vi "Command Intake Cube.vi"(7 "Startup":bool, 9 "Timeout":u32, 11 "Speed":dbl) -> (3 "Output":dbl, 4 "Reinit":bool, 6 "Completed":bool)   [LabVIEW 2017]
uses:
  Command Execution State.ctl
  Intake/Intake Globals.vi
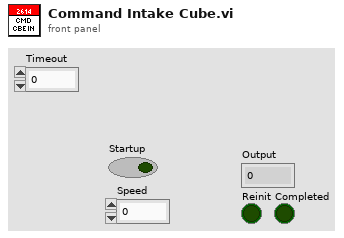
[diagram p1: front panel]
types:
  T1 = typedef "Command Execution State.ctl" = enum16{"Initialize", "Execute", "Finish"}
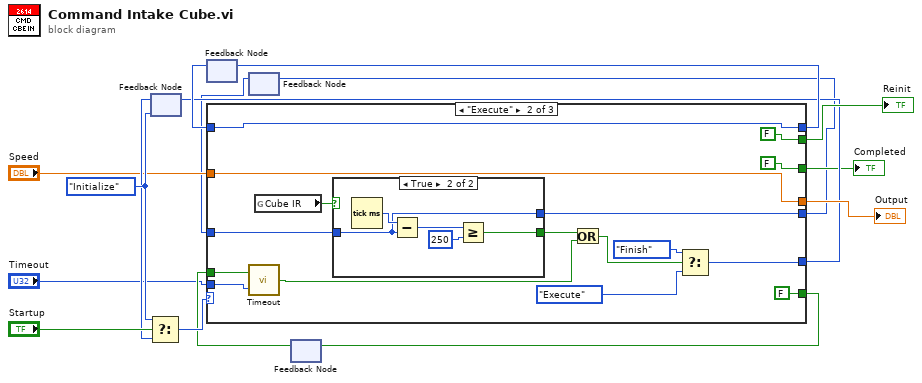
[diagram p0: block diagram]
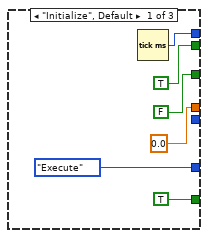
[diagram p2: hidden frame]
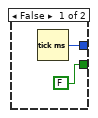
[diagram p3: hidden frame]
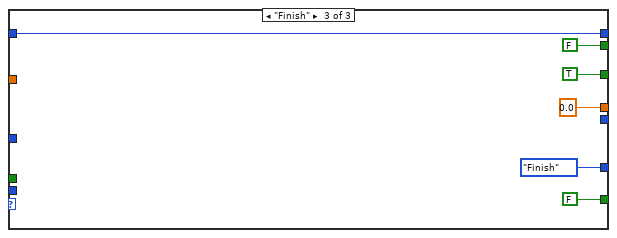
[diagram p4: hidden frame]
diagram:
  w13 = Command_Execution_State."Initialize" ("Play State")
  n1 = feedback #1(w13) -> (w12:T1)
  n2 = Select(t=w13, s="Startup", f=w12) -> (s? t:f=w14:T1)
  n3 = feedback #2() -> (w15:u32)  [unwired: 1 in]
  n4 = feedback #3() -> (w4:u32)  [unwired: 1 in]
  n5 = feedback #4() -> (w2:bool)  [unwired: 1 in]
  n6 = case shown="\"Execute\"" w14 {
    tunnel: w15 -> [_ w38 w47]
    tunnel: "Speed" -> [_ w32 _]
    tunnel: [w22 w38 w47] -> w10
    tunnel: [TRUE FALSE FALSE] -> w9
    tunnel: [0.0 w32 0.0] -> w8
    tunnel: [Command_Execution_State."Execute" ("Play State") w35 Command_Execution_State."Finish" ("Play State")] -> w7
    tunnel: [FALSE FALSE TRUE] -> w6
    tunnel: [_ w30 _] -> w5
    tunnel: w4 -> [_ w29 _]
    tunnel: w2 -> [_ w25 _]
    tunnel: [TRUE FALSE FALSE] -> w3
    tunnel: "Timeout" -> [_ w24 _]
    frame "Initialize", Default {
      n7 = Tick Count (ms)() -> (millisecond timer value=w22:u32)
    }
    frame "Execute" {
      n8 = call "Timeout.vi"("Timeout"=w24, "Initialize"=w25) -> ("Timed Out?"=w26:bool)
      n9 = global read "Intake Globals.vi" "Cube IR"() -> (w31:bool)
      n10 = case shown="True" w31 {
        tunnel: [w40 w43] -> w30
        tunnel: w29 -> [_ w43]
        tunnel: [FALSE w41] -> w28
        frame False {
          n11 = Tick Count (ms)() -> (millisecond timer value=w40:u32)
        }
        frame True {
          n12 = Tick Count (ms)() -> (millisecond timer value=w44:u32)
          n13 = Subtract(x=w44, y=w43) -> (x-y=w45:u32)
          n14 = Greater Or Equal?(x=w45, y=u32 250) -> (x >= y?=w41:bool)
        }
      }
      n15 = Or(x=w28, y=w26) -> (x .or. y?=w27:bool)
      n16 = Select(t=Command_Execution_State."Finish" ("Play State"), s=w27, f=Command_Execution_State."Execute" ("Play State")) -> (s? t:f=w35:T1)
    }
    frame "Finish" {
    }
  }
  "Output" <- w8
  "Reinit" <- w9
  "Completed" <- w6
  n17 = feedback-in #1(w7) -> ()
  n18 = feedback-in #2(w10) -> ()
  n19 = feedback-in #3(w5) -> ()
  n20 = feedback-in #4(w3) -> ()
